vi "run.create.vi"(8 "error in":errorcluster, 11 "Client in":refnum<class "Client.lvclass">) -> (0 "error out":errorcluster, 3 "Client out":refnum<class "Client.lvclass">)   [LabVIEW 2020, in "Client.lvclass"]
doc: "Creates a new run in Nominal with a name, start time, and optional description and end time, and returns a handle to it."
uses:
  Client.lvclass
  client.lvlib
panel:
  out "out_run out":i32
  in  "has_end":bool
  in  "start_ms":dbl
  in  "description":string
  in  "name":string
  in  "out_run":i32
  in  "end_ms":dbl
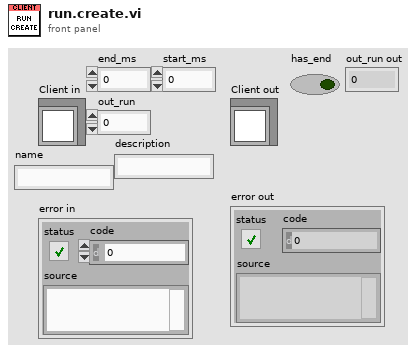
[diagram p1: front panel]
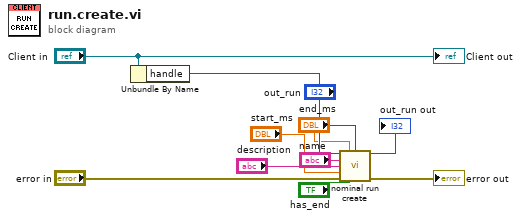
[diagram p0: block diagram]
diagram:
  n1 = Unbundle By Name("Client in") -> ("handle"=w9:i32)
  n2 = call "nominal run create.vi"("client"=w9, "end_ms"="end_ms", "out_run"="out_run", "name"="name", "description"="description", "start_ms"="start_ms", "error in (no error)"="error in", "has_end"="has_end") -> ("out_run out"=→"out_run out":i32, "error out"=→"error out":errorcluster)  [unwired: 5 in, 1 out]
  "Client out" <- "Client in"
